vi "SAturated Sin Amplitude test.vi"() -> ()   [LabVIEW 2017]
uses:
  <vilib>/measure/mascope.llb/Amplitude and Levels 1 chan.vi
  <vilib>/measure/NI_MAPro.lvlib
  <vilib>/measure/NI_MABase.lvlib
  <vilib>/measure/matone.llb/Extract Single Tone Information 1 Chan.vi
panel:
  out "I RMS":dbl
  in  "Scaling":dbl
  out "cal":dbl
  out "low state level":dbl format="%.2g"
  out "high state level":dbl format="%.2g"
  in  "Phase":dbl
  out "Calc Ampl":dbl
  out "Sat. Ind":u64
  out "1/2 Period":i32
  out "Falling":i32
  out "Rising":i32
  in  "Fit Gain":dbl
  out "e 2":waveform(dbl)(graph)
  out "detected phase (deg)":dbl format="%.2p"
  out "detected frequency":dbl format="%.2p"
  out "exported signals":T1 {"exported spectrum (dB)"."dB Spectrum (Hann)" format="%.2p"; "exported spectrum (dB)"."df" format="%.2p"; "exported spectrum (dB)"."f0" format="%.2p"}
  out "detected amplitude":dbl format="%.2p"
  in  "Gain":dbl=10.0 format="%#_13g"
  out "e":dbl[](graph)
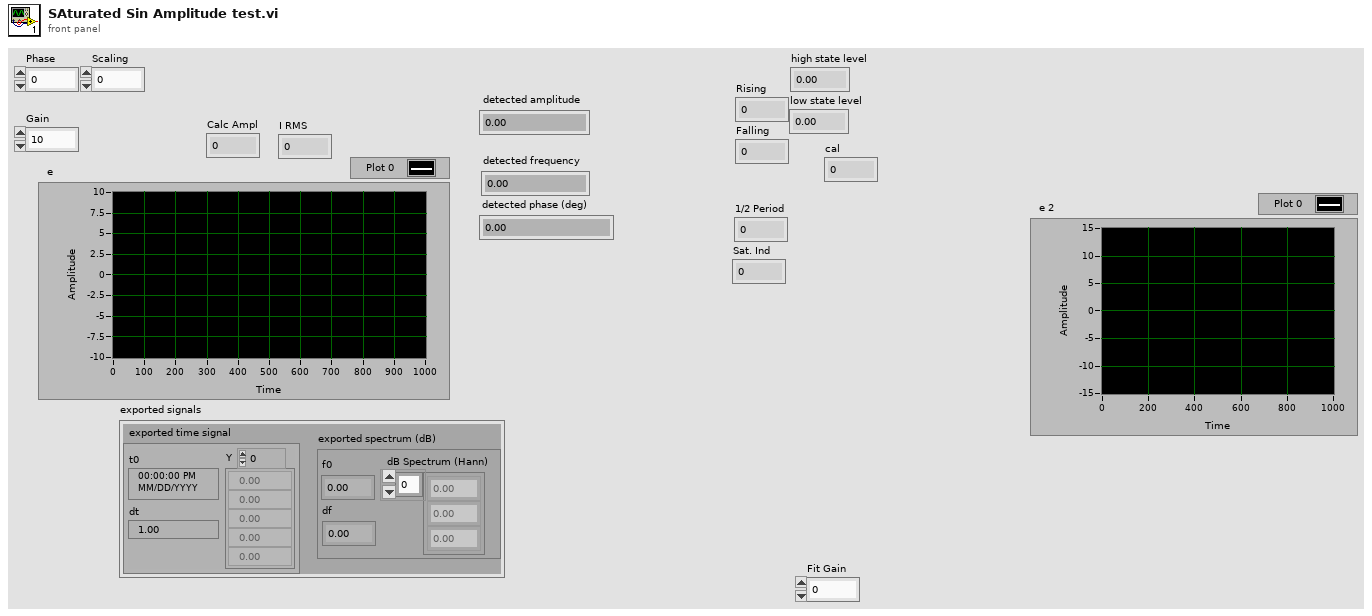
[diagram p1: front panel]
types:
  T1 = cluster{"exported time signal":waveform(dbl), "exported spectrum (dB)":cluster{"f0":dbl, "df":dbl, "dB Spectrum (Hann)":dbl[]}}
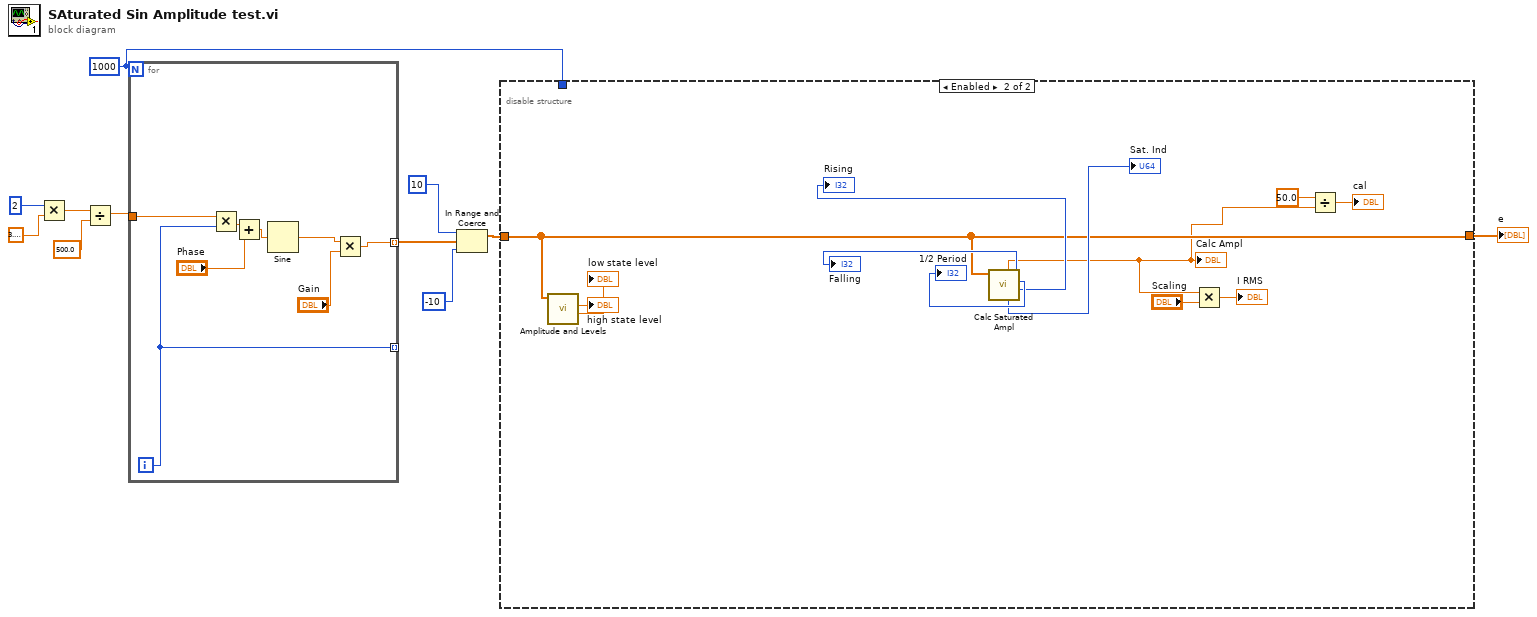
[diagram p0: block diagram]
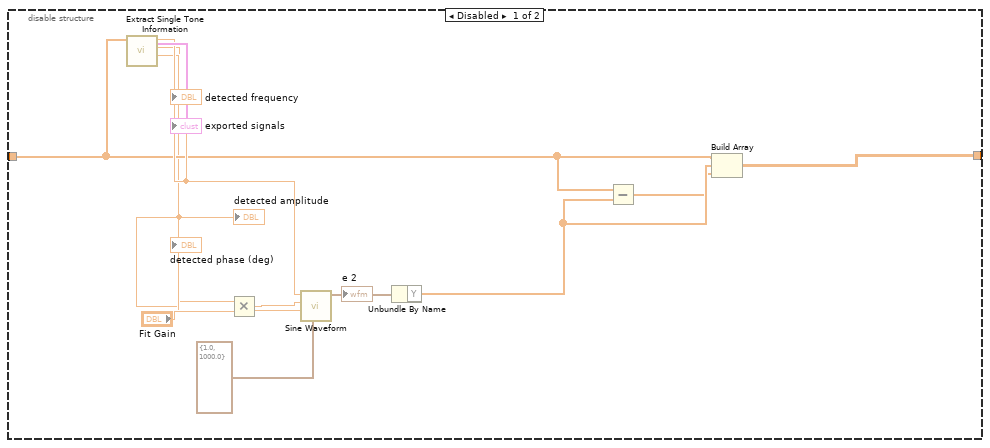
[diagram p2: hidden frame]
diagram:
  w1 = 1000
  n1 = Multiply(x=2, y=3.141592653589793) -> (x*y=w9:dbl)
  n2 = Divide(x=w9, y=500.0) -> (x/y=w8:dbl)
  n3 = for {
    N: w1 -> [_]
    tunnel: w8 -> [w19]
    tunnel: [w16] -> w4 mode=indexing
    tunnel: [w15] -> _ mode=indexing
    i -> [w15]
    n4 = Multiply(x=w19, y=w15) -> (x*y=w14:dbl)
    n5 = Add(x=w14, y="Phase") -> (x+y=w13:dbl)
    n6 = Sine(x=w13) -> (sin(x)=w18:dbl)
    n7 = Multiply(x=w18, y="Gain") -> (x*y=w16:dbl)
  }
  n8 = In Range and Coerce(upper limit=10, x=w4, lower limit=-10) -> (coerced(x)=w3:dbl[])  [unwired: 1 out]
  n9 = disable-structure shown="Enabled" {
    disable-tunnel: w3 -> [w27 w39]
    disable-tunnel: [w25 w39] -> w2
    disable-tunnel: w1 -> [_ _]
    frame Disabled {
      n10 = call-poly <vilib>:"Extract Single Tone Information.vi"("time signal in"=w27) -> ("detected phase (deg)"=w22:dbl, "detected amplitude"=w21:dbl, "detected frequency"=w30:dbl, "exported signals"=→"exported signals":T1)  [unwired: 5 in, 2 out]
      "detected amplitude" <- w21
      "detected frequency" <- w30
      "detected phase (deg)" <- w22
      n11 = Multiply(x=w21, y="Fit Gain") -> (x*y=w20:dbl)
      n12 = call <vilib>:"Sine Waveform.vi"("sampling info"=cluster{"Fs":dbl, "#s":dbl} {"Fs"=1.0, "#s"=1000.0}, "phase"=w22, "amplitude"=w20, "frequency"=w30) -> ("signal out"=w28:waveform(dbl))  [unwired: 6 in, 1 out]
      "e 2" <- w28
      n13 = Unbundle By Name(w28) -> ("Y"=w26:dbl[])
      n14 = Subtract(x=w27, y=w26) -> (x-y=w24:dbl[])
      n15 = Build Array(w27, w26, w24) -> (w25:dbl[][])
    }
    frame Enabled {
      n16 = call-poly <vilib>:"Amplitude and Levels.vi"("signal in"=w39) -> ("low state level"=→"low state level":dbl, "high state level"=→"high state level":dbl)  [unwired: 7 in, 2 out]
      n17 = call "Calc Saturated Ampl.vi"("Waveform"=w39) -> ("Rising"=→"Rising":i32, "1/2 Period"=→"1/2 Period":i32, "Falling"=→"Falling":i32, "Sat. Ind"=→"Sat. Ind":u64, "Peak Amplitude"=w34:dbl)  [unwired: 5 in, 1 out]
      "Calc Ampl" <- w34
      n18 = Multiply(x=w34, y="Scaling") -> (x*y=→"I RMS":dbl)
      n19 = Divide(x=50.0, y=w34) -> (x/y=→"cal":dbl)
    }
  }
  "e" <- w2
